vi "Get Document Type.vi"(8 "error in (no error)":errorcluster, 11 "Document API in":refnum<class "Document API.lvclass">) -> (0 "error out":errorcluster, 2 "Document Type":T1, 3 "Document API out":refnum<class "Document API.lvclass">)   [LabVIEW 2017, in "Document API.lvlib" / "Document API.lvclass"]
uses:
  Document API.lvclass
  Document Type.ctl
  Document API.lvclass/Document API.ctl
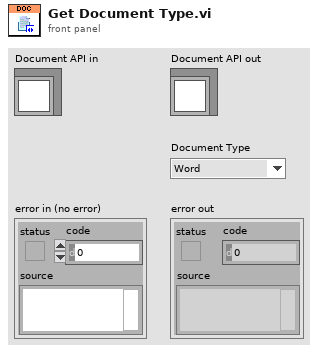
[diagram p1: front panel]
types:
  T1 = typedef "Document API.lvlib/Document API.lvclass/Document Type.ctl" = enum16{"Word", "Excel", "Undefined"}
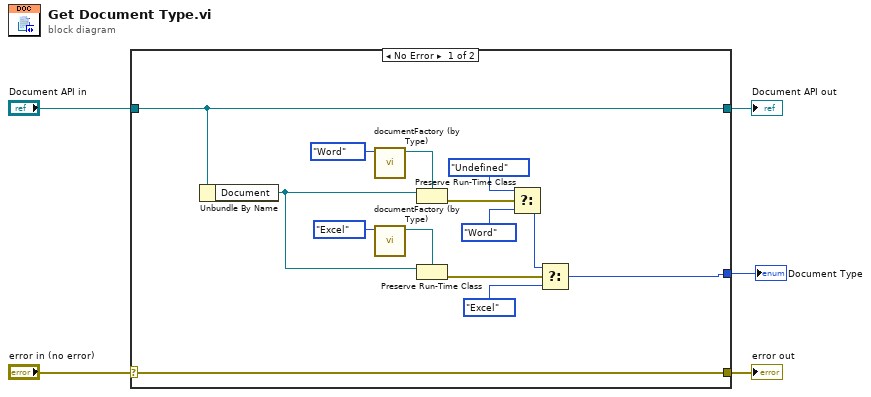
[diagram p0: block diagram]
diagram:
  n1 = case shown="No Error" "error in (no error)" {
    selector: "error in (no error)" -> [w19 w21]
    tunnel: [w19 w21] -> w4
    tunnel: [w18 w20] -> w2
    tunnel: "Document API in" -> [w18 w20]
    tunnel: [w6 _] -> w1
    frame No Error {
      n2 = Unbundle By Name(w18) -> ("Document"=w13:refnum<class "npoiDocument.lvclass">)
      n3 = call "documentFactory (by Type).vi"("Document Type"=Document_Type."Word") -> ("npoiDocument out"=w16:refnum<class "npoiDocument.lvclass">)  [unwired: 9 in, 1 out]
      n4 = call "documentFactory (by Type).vi"("Document Type"=Document_Type."Excel") -> ("npoiDocument out"=w14:refnum<class "npoiDocument.lvclass">)  [unwired: 9 in, 1 out]
      n5 = Preserve Run-Time Class(object in=w13, 2:w16) -> (error out=w12:errorcluster)  [unwired: 1 in, 1 out]
      n6 = Preserve Run-Time Class(object in=w13, 2:w14) -> (error out=w11:errorcluster)  [unwired: 1 in, 1 out]
      n7 = Select(t=Document_Type."Undefined", s=w12, f=Document_Type."Word" ("Document Type")) -> (s? t:f=w9:T1)
      n8 = Select(t=w9, s=w11, f=Document_Type."Excel" ("Document Type")) -> (s? t:f=w6:T1)
    }
    frame Error {
    }
  }
  "error out" <- w4
  "Document API out" <- w2
  "Document Type" <- w1
